vi "Boolean Assert Test.vi"(11 "Data In":bool) -> (3 "Data Out":bool)   [LabVIEW 2016]
uses:
  Core/Assert API Components/Failure Actions.ctl
  Core/Assert API Components/VI References.ctl
  Core/Assert API Components/Assert API Components.lvlib
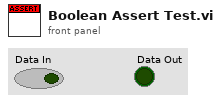
[diagram p1: front panel]
types:
  T1 = typedef "Assert API Components.lvlib/VI References.ctl" = cluster{"Calling VI Ref":refnum<vi>, "Assert VI Ref":refnum<vi>}
  T2 = typedef "Assert API Components.lvlib/Failure Actions.ctl" = enum16{"None", "Log To File", "Pause Execution", "Abort Execution"}
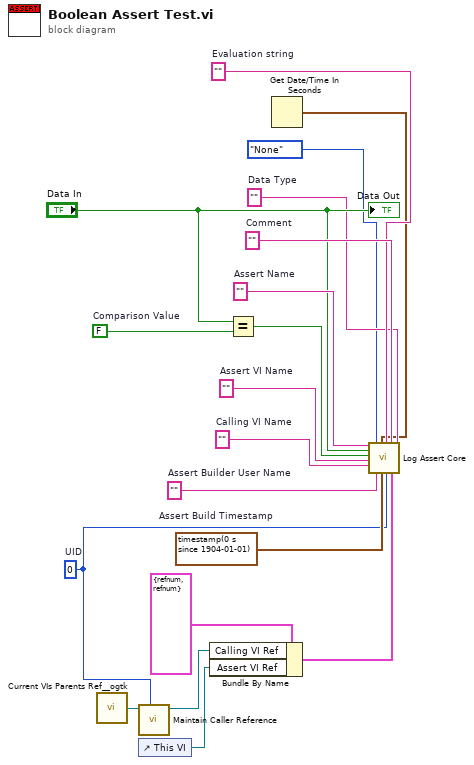
[diagram p0: block diagram]
diagram:
  w1 = 0  # UID
  w7 = ""  # Assert VI Name
  w8 = ""  # Calling VI Name
  w9 = timestamp(0 s since 1904-01-01)  # Assert Build Timestamp
  w10 = ""  # Assert Builder User Name
  w11 = ""  # Data Type
  w18 = ""  # Comment
  w17 = ""  # Evaluation string
  w19 = ""  # Assert Name
  w15 = FALSE  # Comparison Value
  n1 = call <userlib>:"Current VIs Parents Ref__ogtk.vi"() -> ("Calling VI's Reference"=w2:refnum<vi>)  [unwired: 2 in]
  n2 = call "Maintain Caller Reference.vi"("UID"=w1, "VI in"=w2) -> ("VI out"=w3:refnum<vi>)  [unwired: 9 in]
  n3 = control-ref of="This VI"() -> (w12:refnum<vi>)
  n4 = Bundle By Name(cluster=T1 {"Calling VI Ref"=refnum, "Assert VI Ref"=refnum} ("VI References"), "Calling VI Ref"=w3, "Assert VI Ref"=w12) -> (w13:T1)
  n5 = Equal?(x="Data In", y=w15) -> (x = y?=w14:bool)
  n6 = Get Date/Time In Seconds() -> (seconds since 1Jan1904=w5:timestamp)
  n7 = call "Log Assert Core.vi"("Assert Name"=w19, "Data Value"="Data In", "Status"=w14, "Assert VI Name"=w7, "Calling VI Name"=w8, "Failure Action"=Failure_Actions."None" ("Default Failure Action"), "Assert Builder User Name"=w10, "Last Update"=w5, "Assert Build Timestamp"=w9, "Evaluation String"=w17, "Assert VI UID"=w1, "Comment"=w18, "VI References"=w13, "Data Type"=w11) -> ()  [unwired: 6 in]
  "Data Out" <- "Data In"
